vi "oax_Get All Data File Name.vi"() -> (0 "error out":errorcluster, 3 "file names":string[](array[string]))   [LabVIEW 2017]
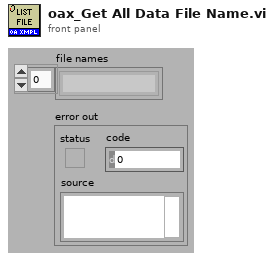
[diagram p1: front panel]
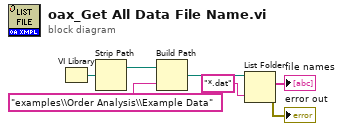
[diagram p0: block diagram]
diagram:
  n1 = VI Library() -> (path=w2:path)
  n2 = Strip Path(path=w2) -> (stripped path=w1:path)  [unwired: 1 out]
  n3 = Build Path(base path=w1, name or relative path="examples\\Order Analysis\\Example Data") -> (appended path=w6:path)
  n4 = List Folder(path=w6, pattern="*.dat") -> (filenames=→"file names":string[], error out=→"error out":errorcluster)  [unwired: 2 in, 2 out]
